vi "2-Position Solenoid Control.vi"(6 "Sensor Analog Status":sgl format="%#_13g", 7 "Sensor Digital Status":bool, 9 "Feedback":T5, 10 "Action":T4(ring), 11 "PneumaticsDevRefIn":T1={"Pneumatic State Reference"=refnum, "SolenoidDevRef"={"DevStatus"={"status"=FALSE, "code"=0, "source"=""}, "Pneumatics Control Module"=0, "Forward Solenoid Channel"=enum."Invalid", "Reverse Solenoid Channel"=enum."Invalid"}, "Pneumatic Configuration reference"=refnum}) -> (1 "Action Complete":bool, 2 "Forward":bool, 3 "PneumaticsDevRefOut":T1={"Pneumatic State Reference"=refnum, "SolenoidDevRef"={"DevStatus"={"status"=FALSE, "code"=0, "source"=""}, "Pneumatics Control Module"=0, "Forward Solenoid Channel"=enum."Invalid", "Reverse Solenoid Channel"=enum."Invalid"}, "Pneumatic Configuration reference"=refnum})   [LabVIEW 2015]
uses:
  <userlib>/836-Library/Pneumatics/Common/Feedback Typedef.ctl
  <userlib>/836-Library/Pneumatics/Pneumatics/836_PneumaticsDevRef.ctl
  <userlib>/836-Library/Pneumatics/Pneumatics/Pneumatic State.ctl
  <userlib>/836-Library/Pneumatics/Pneumatics/StateMachine.ctl
  <vilib>/Rock Robotics/WPI/Solenoid/WPI_SolenoidDevRef.ctl
  <vilib>/Rock Robotics/WPI/Solenoid/WPI_SolenoidChannel.ctl
  <userlib>/836-Library/Pneumatics/Pneumatics/Pneumatic Configuration.ctl
  <vilib>/Rock Robotics/WPI/Solenoid/WPI_SolenoidValue.ctl
  <vilib>/Rock Robotics/WPI/Solenoid/WPI_SolenoidSetEnum.vi
panel:
  out "error IO":errorcluster
  out "Error Out":errorcluster
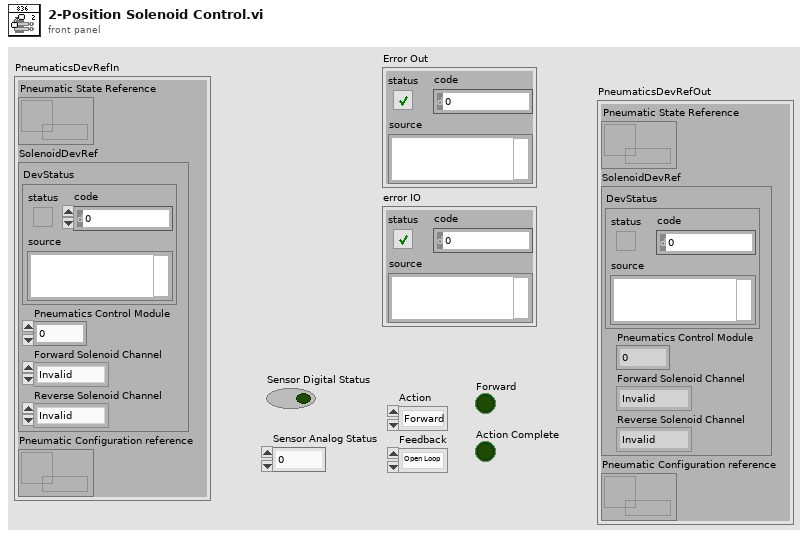
[diagram p1: front panel]
types:
  T1 = typedef "836_PneumaticsDevRef.ctl" = cluster{"Pneumatic State Reference":refnum<data-value>, "SolenoidDevRef":T2, "Pneumatic Configuration reference":refnum<data-value>}
  T2 = typedef "WPI_SolenoidDevRef.ctl" = cluster{"DevStatus":errorcluster, "Pneumatics Control Module":u8, "Forward Solenoid Channel":T3, "Reverse Solenoid Channel":T3}
  T3 = typedef "WPI_SolenoidChannel.ctl" = enum8{"Solenoid 0", "Solenoid 1", "Solenoid 2", "Solenoid 3", "Solenoid 4", "Solenoid 5", "Solenoid 6", "Solenoid 7", "Invalid"}
  T4 = enum16{"Forward", "Back", "Toggle", "Status", "Off"}
  T5 = typedef "Feedback Typedef.ctl" = enum16{"Open Loop", "Analog", "Digital", "Timed", "Digital Timeout"}
  T6 = typedef "WPI_SolenoidValue.ctl" = enum16{"Off", "On", "Forward", "Reverse"}
  T7 = typedef "StateMachine.ctl" = enum8{"Status", "Forward", "Back", "Toggle", "Timed Forward", "Timed Back", "Analog Forwad", "Analog Back", "Digital Forward", "Digital Back", "Off", "Float", "Digital Forward Timeout", "Digital Back Timeout"}
  T8 = typedef "Pneumatic State.ctl" = cluster{"Position":bool, "Initialize":bool, "Current State":T7, "Multiuse Timer A":u32, "Multiuse Timer B":u32}
  T9 = typedef "Pneumatic Configuration.ctl" = cluster{"Time Forward (ms)":u32, "Time Back (ms)":u32, "Digital Forward Time (ms)":u32, "Digital Backward Time (ms)":u32, "Analog Forward Settling Time (ms)":u32, "Analog Backward Settling Time (ms)":u32, "Analog Forward Threshold":sgl, "Analog Backward Threshold":sgl}
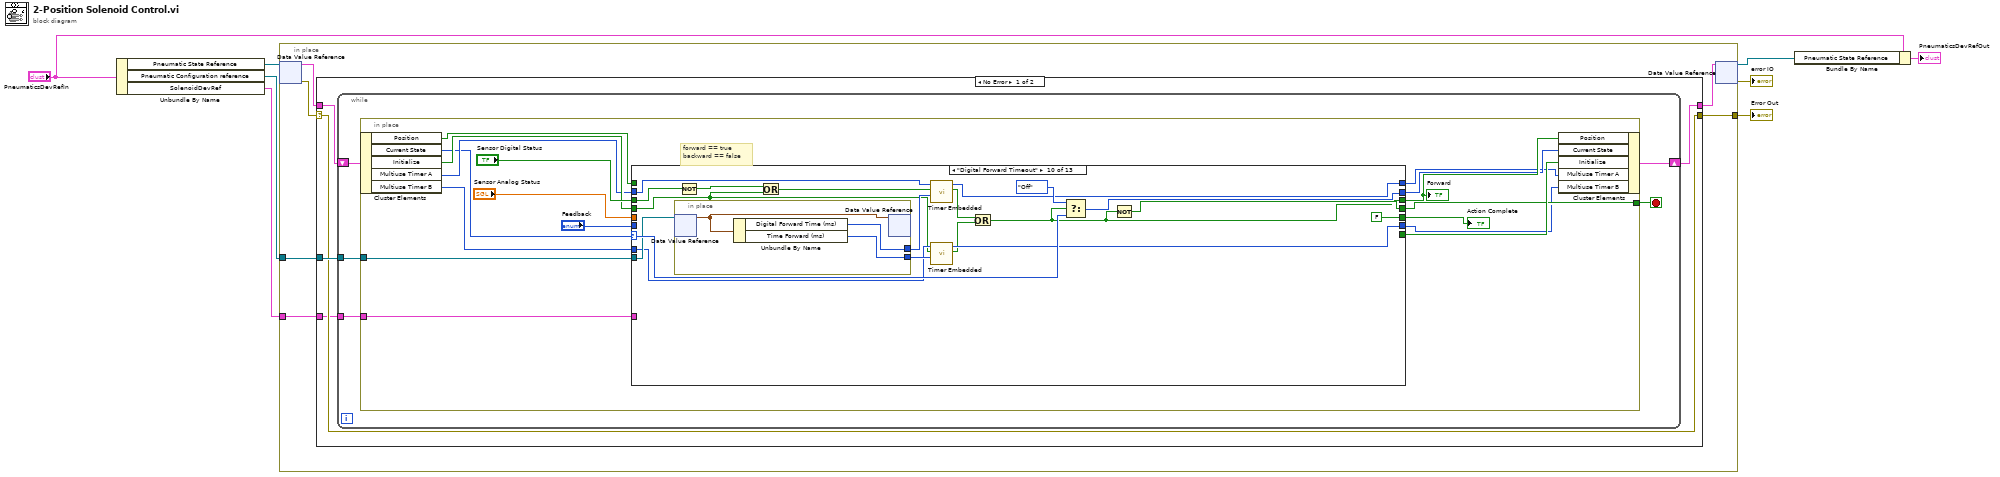
[diagram p0: block diagram]
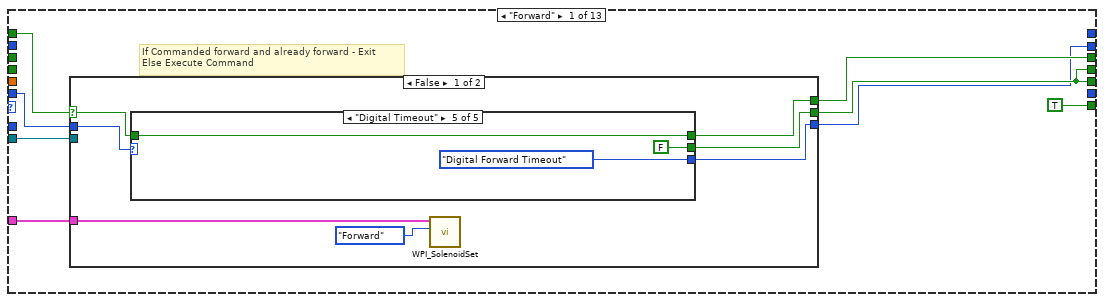
[diagram p2: hidden frame]
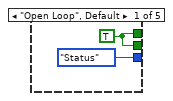
[diagram p3: hidden frame]
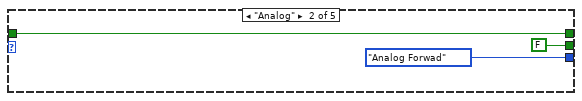
[diagram p4: hidden frame]
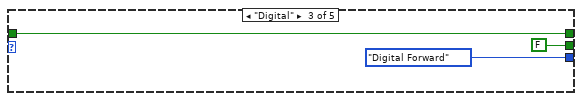
[diagram p5: hidden frame]
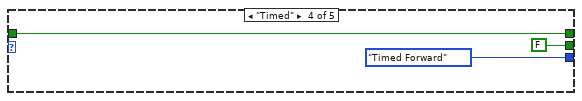
[diagram p6: hidden frame]
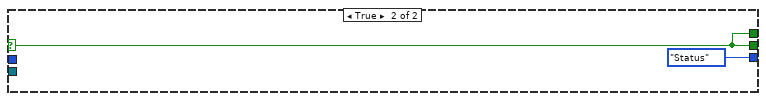
[diagram p7: hidden frame]
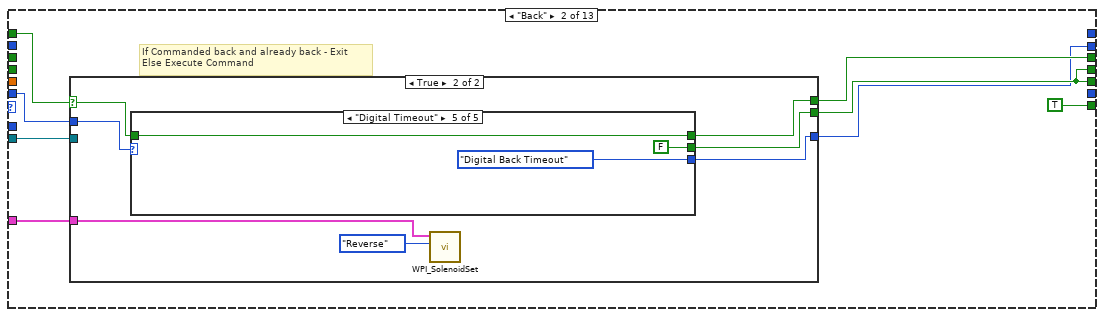
[diagram p8: hidden frame]
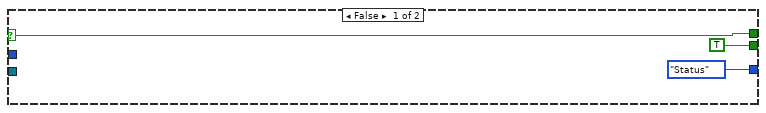
[diagram p9: hidden frame]
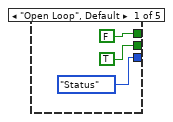
[diagram p10: hidden frame]
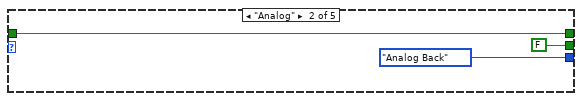
[diagram p11: hidden frame]
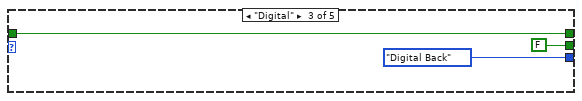
[diagram p12: hidden frame]
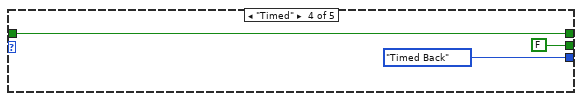
[diagram p13: hidden frame]
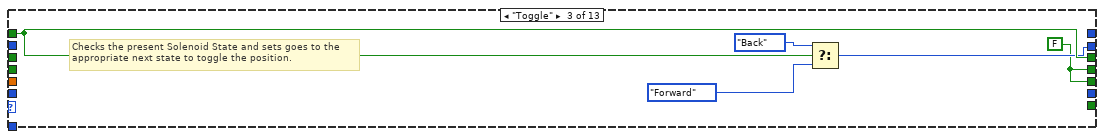
[diagram p14: hidden frame]
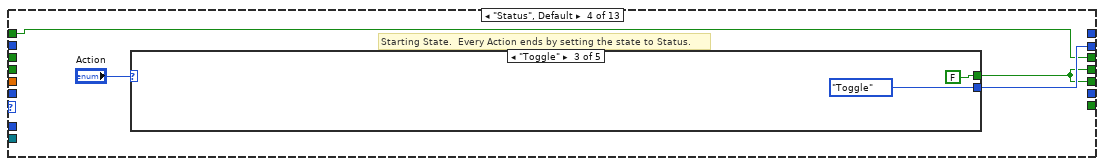
[diagram p15: hidden frame]
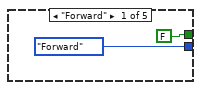
[diagram p16: hidden frame]
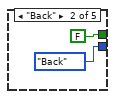
[diagram p17: hidden frame]
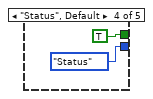
[diagram p18: hidden frame]
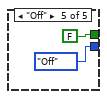
[diagram p19: hidden frame]
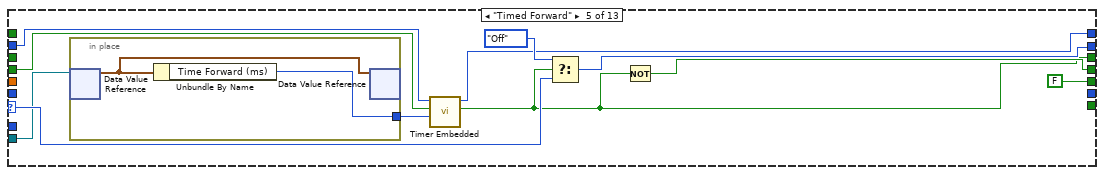
[diagram p20: hidden frame]
diagram:
  n1 = Unbundle By Name("PneumaticsDevRefIn") -> ("Pneumatic State Reference"=w8:refnum<data-value>, "Pneumatic Configuration reference"=w7:refnum<data-value>, "SolenoidDevRef"=w1:T2)
  n2 = in-place {
    in-place-border: w7 -> [w13]
    in-place-border: [w10] -> w3
    in-place-border: w1 -> [w9]
    n3 = in-place-dvr #1(w8) -> (w14:T8, w11:errorcluster)
    n4 = case shown="No Error" w11 {
      selector: w11 -> [w17 w269]
      tunnel: w14 -> [w19 w270]
      tunnel: w13 -> [w18 _]
      tunnel: [w16 w270] -> w12
      tunnel: [w17 w269] -> w10
      tunnel: w9 -> [w15 _]
      frame No Error {
        n5 = while {
          tunnel: w18 -> [w23]
          shift-right: [w21] -> w16
          shift-left: w19 -> [w24]
          tunnel: w15 -> [w20]
          stop <- w22 stop-if-true
          n6 = in-place {
            in-place-border: w23 -> [w33]
            in-place-border: [w29] -> w22
            in-place-border: w20 -> [w27]
            # "forward == true\nbackward == false"
            n7 = in-place-cluster #2(w24) -> ("Position"=w37:bool, "Current State"=w31:T7, "Initialize"=w36:bool, "Multiuse Timer A"=w32:u32, "Multiuse Timer B"=w26:u32)
            n8 = case shown="\"Digital Forward Timeout\"" w31 {
              selector: w31 -> [_ _ _ _ w133 w146 w165 w175 w202 w223 w231 w247 _]
              tunnel: [w47 w78 w106 w112 w131 w140 w163 w172 w199 w220 w228 w244 w266] -> w29
              tunnel: "Feedback" -> [w49 w80 _ _ _ _ _ _ _ _ _ _ _]
              tunnel: w37 -> [w45 w77 w109 w113 _ _ _ _ _ _ _ _ w267]
              tunnel: [w48 w79 w109 w113 w126 w140 w157 w172 w193 w206 w228 w244 w267] -> w35
              tunnel: "Sensor Digital Status" -> [_ _ _ _ _ _ _ _ w191 w208 w239 w259 _]
              tunnel: [w46 w76 w107 w114 w134 w149 w168 w186 w203 w224 w240 w260 StateMachine."Status"] -> w34
              tunnel: "Sensor Analog Status" -> [_ _ _ _ _ _ w167 w185 _ _ _ _ _]
              tunnel: w36 -> [_ _ _ _ w128 w141 w155 w182 w192 w209 w237 w253 _]
              tunnel: [w47 w78 w106 w112 FALSE FALSE FALSE FALSE FALSE FALSE FALSE FALSE w266] -> w38
              tunnel: w32 -> [_ _ _ _ w129 w142 w160 w178 w196 w212 w233 w251 _]
              tunnel: [_ _ _ _ w125 w143 w159 w177 w194 w211 w232 w248 _] -> w28
              tunnel: w33 -> [w44 w75 _ _ w130 w139 w162 w181 w198 w219 w236 w257 _]
              tunnel: [TRUE TRUE _ _ _ _ _ _ _ _ _ _ _] -> w30
              tunnel: w27 -> [w42 w73 _ _ _ _ _ _ _ _ _ _ w265]
              tunnel: w26 -> [_ _ _ _ _ _ _ _ _ w217 _ w254 _]
              tunnel: [_ _ _ _ _ _ _ _ _ w216 _ w255 _] -> w25
              frame "Forward" {
                # "If Commanded forward and already forward - Exit\nElse Execute Command"
                n9 = case shown="False" w45 {
                  selector: w45 -> [w52 w71]
                  tunnel: w49 -> [w56 _]
                  tunnel: [w55 w71] -> w48
                  tunnel: [w54 w71] -> w47
                  tunnel: [w53 StateMachine."Status"] -> w46
                  tunnel: w44 -> [_ _]
                  tunnel: w42 -> [w51 _]
                  frame False {
                    n10 = case shown="\"Digital Timeout\"" w56 {
                      tunnel: [w57 FALSE FALSE FALSE FALSE] -> w54
                      tunnel: [StateMachine."Status" StateMachine."Analog Forwad" StateMachine."Digital Forward" StateMachine."Timed Forward" StateMachine."Digital Forward Timeout"] -> w53
                      tunnel: w52 -> [_ w59 w62 w65 w68]
                      tunnel: [w57 w59 w62 w65 w68] -> w55
                      frame "Open Loop", Default {
                        w57 = TRUE
                      }
                      frame "Analog" {
                      }
                      frame "Digital" {
                      }
                      frame "Timed" {
                      }
                      frame "Digital Timeout" {
                      }
                    }
                    n11 = call-poly <vilib>:"WPI_SolenoidSet.vi"("Value"=WPI_SolenoidValue."Forward" ("Value 3"), "SolenoidDevRef"=w51) -> ()  [unwired: 8 in, 2 out]
                  }
                  frame True {
                  }
                }
              }
              frame "Back" {
                # "If Commanded back and already back - Exit\nElse Execute Command"
                n12 = case shown="True" w77 {
                  selector: w77 -> [w81 w86]
                  tunnel: w80 -> [_ w90]
                  tunnel: [w81 w89] -> w79
                  tunnel: [TRUE w88] -> w78
                  tunnel: [StateMachine."Status" w87] -> w76
                  tunnel: w75 -> [_ _]
                  tunnel: w73 -> [_ w85]
                  frame False {
                  }
                  frame True {
                    n13 = case shown="\"Digital Timeout\"" w90 {
                      tunnel: [TRUE FALSE FALSE FALSE FALSE] -> w88
                      tunnel: [StateMachine."Status" StateMachine."Analog Back" StateMachine."Digital Back" StateMachine."Timed Back" StateMachine."Digital Back Timeout"] -> w87
                      tunnel: [FALSE w94 w97 w100 w103] -> w89
                      tunnel: w86 -> [_ w94 w97 w100 w103]
                      frame "Open Loop", Default {
                      }
                      frame "Analog" {
                      }
                      frame "Digital" {
                      }
                      frame "Timed" {
                      }
                      frame "Digital Timeout" {
                      }
                    }
                    n14 = call-poly <vilib>:"WPI_SolenoidSet.vi"("Value"=WPI_SolenoidValue."Reverse" ("Value 3"), "SolenoidDevRef"=w85) -> ()  [unwired: 8 in, 2 out]
                  }
                }
              }
              frame "Toggle" {
                w106 = FALSE
                # "Checks the present Solenoid State and sets goes to the\nappropriate next state to toggle the position."
                n15 = Select(t=StateMachine."Back", s=w109, f=StateMachine."Forward") -> (s? t:f=w107:T7)
              }
              frame "Status", Default {
                # "Starting State.  Every Action ends by setting the state to Status."
                n16 = case shown="\"Toggle\"" "Action" {
                  tunnel: [FALSE FALSE FALSE TRUE FALSE] -> w112
                  tunnel: [StateMachine."Forward" StateMachine."Back" StateMachine."Toggle" StateMachine."Status" StateMachine."Off"] -> w114
                  frame "Forward" {
                  }
                  frame "Back" {
                  }
                  frame "Toggle" {
                  }
                  frame "Status", Default {
                  }
                  frame "Off" {
                  }
                }
              }
              frame "Timed Forward" {
                n17 = in-place {
                  in-place-border: [w136] -> w127
                  n18 = in-place-dvr #3(w130) -> (w137:T9)  [unwired: 1 out]
                  n19 = Unbundle By Name(w137) -> ("Time Forward (ms)"=w136:u32)
                  n20 = in-place-dvr #3(w137) -> ()  [unwired: 2 out]
                }
                n21 = call <userlib>:"Timer Embedded.vi"("Time Limit"=w127, "Reset"=w128, "Start Time In"=w129) -> ("Time Limit Passed"=w126:bool, "Start Time Out"=w125:u32)  [unwired: 7 in]
                n22 = Select(t=StateMachine."Off", s=w126, f=w133) -> (s? t:f=w134:T7)
                n23 = Not(x=w126) -> (.not. x?=w131:bool)
              }
              frame "Timed Back" {
                n24 = case shown="True" w141 {
                  tunnel: [w152 w153] -> w143
                  tunnel: w142 -> [w152 _]
                  frame False {
                  }
                  frame True {
                    n25 = Tick Count (ms)() -> (millisecond timer value=w153:u32)
                  }
                }
                n26 = in-place {
                  in-place-border: [w150] -> w138
                  n27 = in-place-dvr #4(w139) -> (w151:T9)  [unwired: 1 out]
                  n28 = Unbundle By Name(w151) -> ("Time Back (ms)"=w150:u32)
                  n29 = in-place-dvr #4(w151) -> ()  [unwired: 2 out]
                }
                n30 = Tick Count (ms)() -> (millisecond timer value=w145:u32)
                n31 = Subtract(x=w145, y=w143) -> (x-y=w148:u32)
                n32 = Less Or Equal?(x=w148, y=w138) -> (x <= y?=w140:bool)
                n33 = Select(t=w146, s=w140, f=StateMachine."Off") -> (s? t:f=w149:T7)
              }
              frame "Analog Forwad" {
                n34 = in-place {
                  in-place-border: [w170] -> w158
                  in-place-border: [w169] -> w161
                  n35 = in-place-dvr #5(w162) -> (w171:T9)  [unwired: 1 out]
                  n36 = Unbundle By Name(w171) -> ("Analog Forward Settling Time (ms)"=w170:u32, "Analog Forward Threshold"=w169:sgl)
                  n37 = in-place-dvr #5(w171) -> ()  [unwired: 2 out]
                }
                n38 = Less?(x=w167, y=w161) -> (x < y?=w156:bool)
                n39 = Or(x=w155, y=w156) -> (x .or. y?=w154:bool)
                n40 = call <userlib>:"Timer Embedded.vi"("Time Limit"=w158, "Reset"=w154, "Start Time In"=w160) -> ("Time Limit Passed"=w157:bool, "Start Time Out"=w159:u32)  [unwired: 7 in]
                n41 = Select(t=StateMachine."Off", s=w157, f=w165) -> (s? t:f=w168:T7)
                n42 = Not(x=w157) -> (.not. x?=w163:bool)
              }
              frame "Analog Back" {
                n43 = in-place {
                  in-place-border: [w188] -> w180
                  in-place-border: [w187] -> w176
                  n44 = in-place-dvr #6(w181) -> (w189:T9)  [unwired: 1 out]
                  n45 = Unbundle By Name(w189) -> ("Analog Backward Threshold"=w188:sgl, "Analog Backward Settling Time (ms)"=w187:u32)
                  n46 = in-place-dvr #6(w189) -> ()  [unwired: 2 out]
                }
                n47 = Greater?(x=w185, y=w180) -> (0:w184:bool)
                n48 = Or(x=w182, y=w184) -> (x .or. y?=w179:bool)
                n49 = call <userlib>:"Timer Embedded.vi"("Time Limit"=w176, "Reset"=w179, "Start Time In"=w178) -> ("Time Limit Passed"=w173:bool, "Start Time Out"=w177:u32)  [unwired: 7 in]
                n50 = Select(t=StateMachine."Off", s=w173, f=w175) -> (s? t:f=w186:T7)
                n51 = Not(x=w173) -> (.not. x?=w172:bool)
              }
              frame "Digital Forward" {
                n52 = in-place {
                  in-place-border: [w204] -> w197
                  n53 = in-place-dvr #7(w198) -> (w205:T9)  [unwired: 1 out]
                  n54 = Unbundle By Name(w205) -> ("Digital Forward Time (ms)"=w204:u32)
                  n55 = in-place-dvr #7(w205) -> ()  [unwired: 2 out]
                }
                n56 = Not(x=w191) -> (.not. x?=w190:bool)
                n57 = Or(x=w190, y=w192) -> (x .or. y?=w195:bool)
                n58 = call <userlib>:"Timer Embedded.vi"("Time Limit"=w197, "Reset"=w195, "Start Time In"=w196) -> ("Time Limit Passed"=w193:bool, "Start Time Out"=w194:u32)  [unwired: 7 in]
                n59 = Select(t=StateMachine."Off", s=w193, f=w202) -> (s? t:f=w203:T7)
                n60 = Not(x=w193) -> (.not. x?=w199:bool)
              }
              frame "Digital Forward Timeout" {
                n61 = in-place {
                  in-place-border: [w226] -> w214
                  in-place-border: [w225] -> w218
                  n62 = in-place-dvr #8(w219) -> (w227:T9)  [unwired: 1 out]
                  n63 = Unbundle By Name(w227) -> ("Digital Forward Time (ms)"=w226:u32, "Time Forward (ms)"=w225:u32)
                  n64 = in-place-dvr #8(w227) -> ()  [unwired: 2 out]
                }
                n65 = Not(x=w208) -> (.not. x?=w207:bool)
                n66 = Or(x=w207, y=w209) -> (x .or. y?=w213:bool)
                n67 = call <userlib>:"Timer Embedded.vi"("Time Limit"=w214, "Reset"=w213, "Start Time In"=w212) -> ("Time Limit Passed"=w210:bool, "Start Time Out"=w211:u32)  [unwired: 7 in]
                n68 = call <userlib>:"Timer Embedded.vi"("Time Limit"=w218, "Reset"=w209, "Start Time In"=w217) -> ("Time Limit Passed"=w215:bool, "Start Time Out"=w216:u32)  [unwired: 7 in]
                n69 = Or(x=w210, y=w215) -> (x .or. y?=w206:bool)
                n70 = Select(t=StateMachine."Off", s=w206, f=w223) -> (s? t:f=w224:T7)
                n71 = Not(x=w206) -> (.not. x?=w220:bool)
              }
              frame "Digital Back" {
                n72 = in-place {
                  in-place-border: [w241] -> w235
                  n73 = in-place-dvr #9(w236) -> (w242:T9)  [unwired: 1 out]
                  n74 = Unbundle By Name(w242) -> ("Digital Backward Time (ms)"=w241:u32)
                  n75 = in-place-dvr #9(w242) -> ()  [unwired: 2 out]
                }
                n76 = Or(x=w239, y=w237) -> (x .or. y?=w234:bool)
                n77 = call <userlib>:"Timer Embedded.vi"("Time Limit"=w235, "Reset"=w234, "Start Time In"=w233) -> ("Time Limit Passed"=w229:bool, "Start Time Out"=w232:u32)  [unwired: 7 in]
                n78 = Select(t=StateMachine."Off", s=w229, f=w231) -> (s? t:f=w240:T7)
                n79 = Not(x=w229) -> (.not. x?=w228:bool)
              }
              frame "Digital Back Timeout" {
                n80 = in-place {
                  in-place-border: [w262] -> w250
                  in-place-border: [w261] -> w252
                  n81 = in-place-dvr #10(w257) -> (w263:T9)  [unwired: 1 out]
                  n82 = Unbundle By Name(w263) -> ("Digital Backward Time (ms)"=w262:u32, "Time Back (ms)"=w261:u32)
                  n83 = in-place-dvr #10(w263) -> ()  [unwired: 2 out]
                }
                n84 = Or(x=w259, y=w253) -> (x .or. y?=w249:bool)
                n85 = call <userlib>:"Timer Embedded.vi"("Time Limit"=w250, "Reset"=w249, "Start Time In"=w251) -> ("Time Limit Passed"=w245:bool, "Start Time Out"=w248:u32)  [unwired: 7 in]
                n86 = call <userlib>:"Timer Embedded.vi"("Time Limit"=w252, "Reset"=w253, "Start Time In"=w254) -> ("Time Limit Passed"=w256:bool, "Start Time Out"=w255:u32)  [unwired: 7 in]
                n87 = Or(x=w245, y=w256) -> (x .or. y?=w243:bool)
                n88 = Select(t=StateMachine."Off", s=w243, f=w247) -> (s? t:f=w260:T7)
                n89 = Not(x=w243) -> (.not. x?=w244:bool)
              }
              frame "Off" {
                w266 = TRUE
                n90 = call-poly <vilib>:"WPI_SolenoidSet.vi"("Value"=WPI_SolenoidValue."Off" ("Value 3"), "SolenoidDevRef"=w265) -> ()  [unwired: 8 in, 2 out]
              }
            }
            "Forward" <- w35
            "Action Complete" <- w38
            n91 = in-place-cluster #2("Position"=w35, "Current State"=w34, "Initialize"=w30, "Multiuse Timer A"=w28, "Multiuse Timer B"=w25) -> (w21:T8)
          }
        }
      }
      frame Error {
      }
    }
    n92 = in-place-dvr #1(w12) -> (w4:refnum<data-value>, →"error IO":errorcluster)
  }
  "Error Out" <- w3
  n93 = Bundle By Name(cluster="PneumaticsDevRefIn", "Pneumatic State Reference"=w4) -> (→"PneumaticsDevRefOut":T1)
